vi "LabVIEW_Arduino-AlsDeLampHetDoetIsHetVIGoed.vi"() -> ()   [LabVIEW 2020]
uses:
  <vilib>/LabVIEW Interface for Arduino/Type Defs/Board Type.ctl
  <vilib>/LabVIEW Interface for Arduino/Type Defs/Connection Type.ctl
  <vilib>/LabVIEW Interface for Arduino/LabVIEW Interface for Arduino.lvlib
panel:
  in  "stop":bool
  in  "Boolean":bool
  # "Pas onderstaande in LIFA_Base aan"
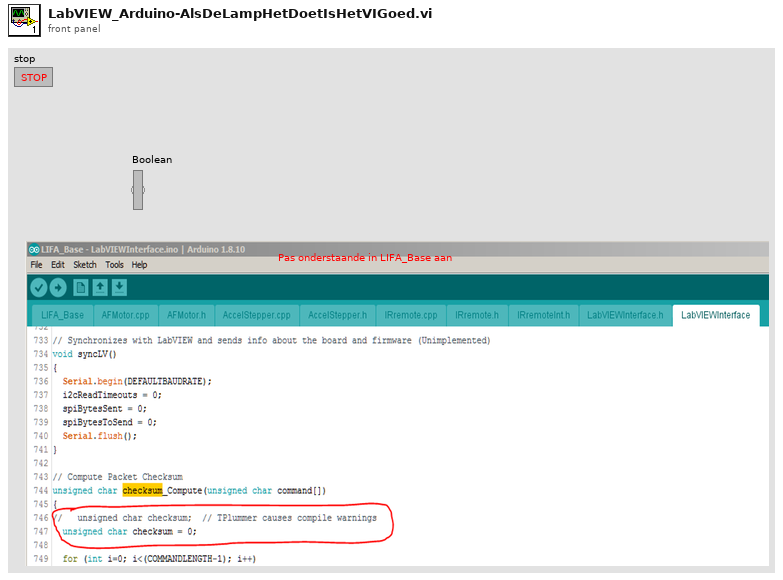
[diagram p1: front panel]
types:
  T1 = typedef "LabVIEW Interface for Arduino.lvlib/Connection Type.ctl" = enum8{"USB / Serial", "XBEE", "BlueSmirf (Bluetooth)"}
  T2 = typedef "LabVIEW Interface for Arduino.lvlib/Board Type.ctl" = enum16{"Uno", "Dimuelanove w/Atmega 328", "Mega 2560"}
  T3 = typedef "LabVIEW Interface for Arduino.lvlib/Arduino Resource.ctl" = cluster{"VISA resource":refnum<visa-resource-name>, "Board Type":T2, "Connection Type":enum8{"USB / Serial"}, "Bytes Per Packet (15)":u8}
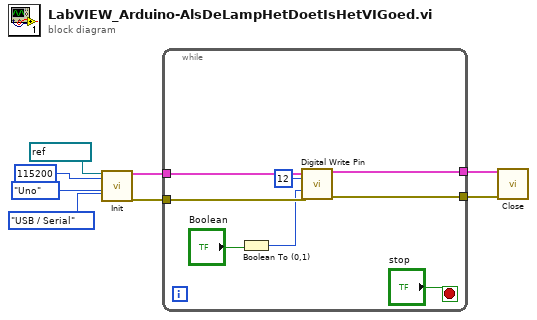
[diagram p0: block diagram]
diagram:
  n1 = call <vilib>:"Init.vi"("VISA resource"=refnum<visa-resource-name> "COM3", "Baud Rate (115200)"=u32 115200, "Board Type (Uno)"=Board_Type."Uno", "Connection Type (USB/Serial)"=Connection_Type."USB / Serial") -> ("Arduino Resource"=w8:T3, "error out"=w6:errorcluster)  [unwired: 14 in]
  n2 = while {
    tunnel: w8 -> [w16]
    tunnel: [w15] -> w7
    tunnel: w6 -> [w14]
    tunnel: [w13] -> w5
    stop <- "stop" stop-if-true
    n3 = Boolean To (0,1)(Boolean="Boolean") -> (0, 1=w10:i16)
    n4 = call <vilib>:"Digital Write Pin.vi"("Arduino Resource"=w16, "Digital I/O Pin (0)"=u8 12, "Value (0)"=w10, "error in"=w14) -> ("Arduino Resource"=w15:T3, "error out"=w13:errorcluster)  [unwired: 10 in]
  }
  n5 = call <vilib>:"Close.vi"("Arduino Resource"=w7, "error in"=w5) -> ()  [unwired: 13 in, 1 out]
